vi "AddDependenciesOfLibrary.vi"(8 "error in (no error)":errorcluster, 9 "LibraryName":string="ModuleA", 10 "Project Path":path=path "E:/sw-deps-monitor/Source/BuildSpecs/Modules/ModuleA.lvproj", 11 "Config Refnum in":T1) -> (0 "error out":errorcluster, 2 "ActualDependencies":string[](array[string]), 3 "Config Refnum out":T1)   [LabVIEW 2023, in "Reusables.lvlib"]
uses:
  Reusables.lvlib
  <vilib>/Utility/config.llb/Config Data RefNum.ctl
  <vilib>/Utility/config.llb/Write Key (String).vi
  <vilib>/Utility/config.llb/NI_LVConfig.lvlib
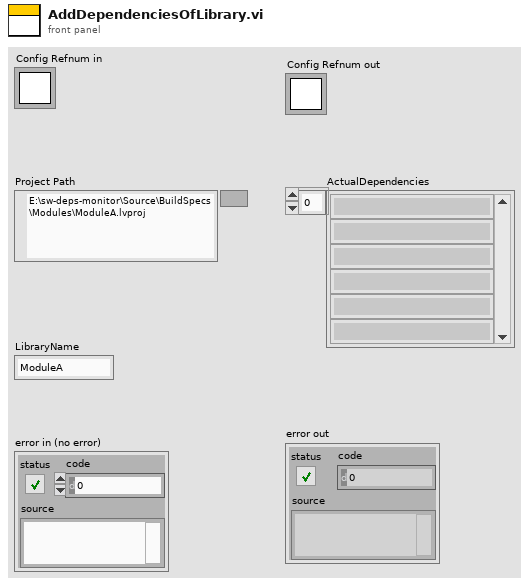
[diagram p1: front panel]
types:
  T1 = typedef "NI_LVConfig.lvlib/Config Data RefNum.ctl" = refnum<k1>
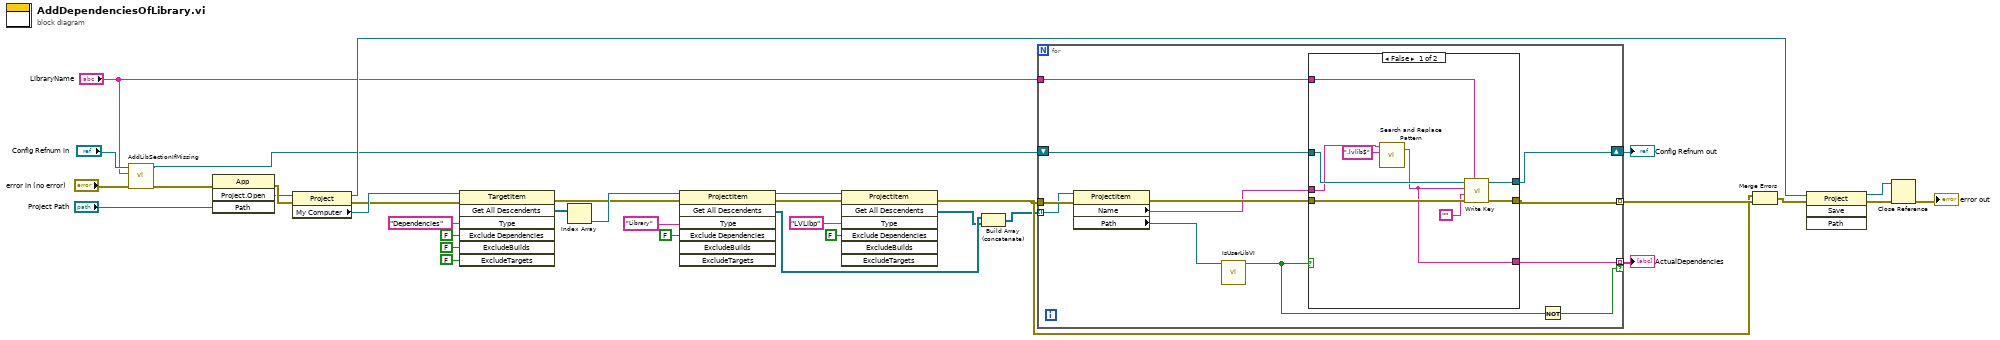
[diagram p0: block diagram]
diagram:
  n1 = call "AddLibSectionIfMissing.vi"("error in (no error)"="error in (no error)", "LibraryName"="LibraryName", "Config Refnum in"="Config Refnum in") -> ("error out"=w5:errorcluster, "Config Refnum out"=w3:T1)  [unwired: 7 in]
  n2 = invoke class="App" method="Project.Open"(error in=w5, "Path"="Project Path") -> (error out=w34:errorcluster, "Project:Open"=w33:refnum<vi>)  [unwired: 2 in, 2 out]
  n3 = property class="Project"(reference=w33, error in=w34) -> (reference out=w18:refnum<vi>, error out=w21:errorcluster, "My Computer"=w27:refnum<vi>)
  n4 = invoke class="TargetItem" method="Get All Descendents"(reference=w27, error in=w21, "Type"="Dependencies", "Exclude Dependencies"=FALSE ("ExcludeDependencies"), "ExcludeBuilds"=FALSE, "ExcludeTargets"=FALSE) -> (error out=w20:errorcluster, "All Descendents"=w23:refnum<vi>[])  [unwired: 1 in, 5 out]
  n5 = Index Array(array=w23) -> (element=w22:refnum<vi>)  [unwired: 1 in]
  n6 = invoke class="ProjectItem" method="Get All Descendents"(reference=w22, error in=w20, "Type"="Library", "Exclude Dependencies"=FALSE ("ExcludeDependencies")) -> (reference out=w13:refnum<vi>, error out=w14:errorcluster, "All Descendents"=w9:refnum<vi>[])  [unwired: 3 in, 4 out]
  n7 = invoke class="ProjectItem" method="Get All Descendents"(reference=w13, error in=w14, "Type"="LVLibp", "Exclude Dependencies"=FALSE ("ExcludeDependencies")) -> (error out=w10:errorcluster, "All Descendents"=w8:refnum<vi>[])  [unwired: 3 in, 5 out]
  n8 = Build Array (concatenate)(w9, w8) -> (w7:refnum<vi>[])
  n9 = for {
    tunnel: w10 -> [w47]
    tunnel: w7 -> [w40] mode=indexing
    tunnel: "LibraryName" -> [w44]
    tunnel: [w41] -> w32 mode=indexing
    shift-right: [w42] -> w31
    shift-left: w3 -> [w46]
    tunnel: [w38] -> w1 mode=indexing if=w36
    n10 = property class="ProjectItem"(reference=w40, error in=w47) -> (error out=w45:errorcluster, "Name"=w43:string, "Path"=w39:path)  [unwired: 1 out]
    n11 = call "IsUserLibVI.vi"("ItemPath"=w39) -> ("IsUserLibVI?"=w37:bool)  [unwired: 10 in]
    n12 = case shown="False" w37 {
      tunnel: w46 -> [w55 w57]
      tunnel: w45 -> [w56 w58]
      tunnel: w44 -> [w54 _]
      tunnel: w43 -> [w51 _]
      tunnel: [w50 w58] -> w41
      tunnel: [w49 w57] -> w42
      tunnel: [w48 _] -> w38
      frame False {
        n13 = call <vilib>:"Search and Replace Pattern.vi"("string"=w51, "regular expression (\"\")"=".lvlib$" ("regular expression (\"\")")) -> ("result string"=w48:string)  [unwired: 3 in, 1 out]
        n14 = call-poly <vilib>:"Write Key.vi"("section"=w54, "error in (no error)"=w56, "value"="", "key"=w48, "refnum"=w55) -> ("error out"=w50:errorcluster, "refnum out"=w49:T1)  [unwired: 4 in, 1 out]
      }
      frame True {
      }
    }
    n15 = Not(x=w37) -> (.not. x?=w36:bool)
  }
  "Config Refnum out" <- w31
  "ActualDependencies" <- w1
  n16 = Merge Errors(w10, w32) -> (w19:errorcluster)
  n17 = invoke class="Project" method="Save"(reference=w18, error in=w19) -> (reference out=w17:refnum<vi>, error out=w16:errorcluster)  [unwired: 2 in, 2 out]
  n18 = Close Reference(reference=w17, error in (no error)=w16) -> (error out=→"error out":errorcluster)
